vi "Build and convert part number.vi"(10 "Digit Array":T1[](array[typedef]), 11 "Unsigned Byte Array":u8[][](array[numeric])) -> (2 "Part Number Found Out":bool, 3 "Part Number Out":i32)   [LabVIEW 2023]
uses:
  Cluster Digit.ctl
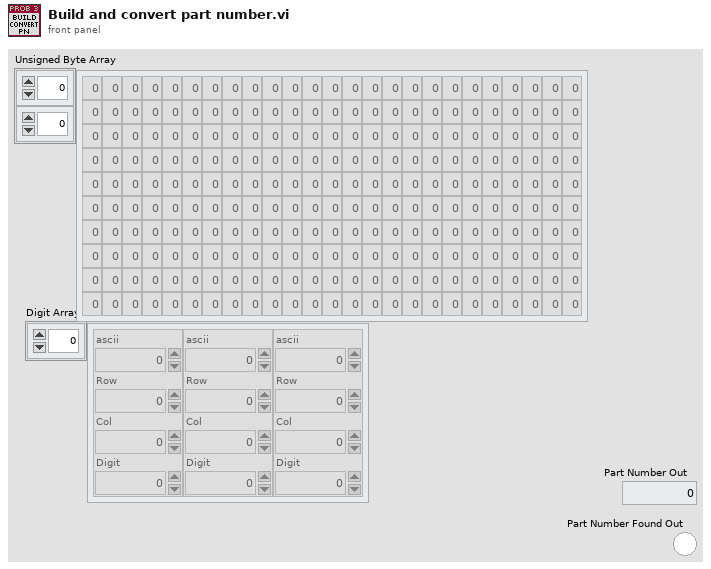
[diagram p1: front panel]
types:
  T1 = typedef "Cluster Digit.ctl" = cluster{"ascii":u8, "Row":i32, "Col":i32, "Digit":i32}
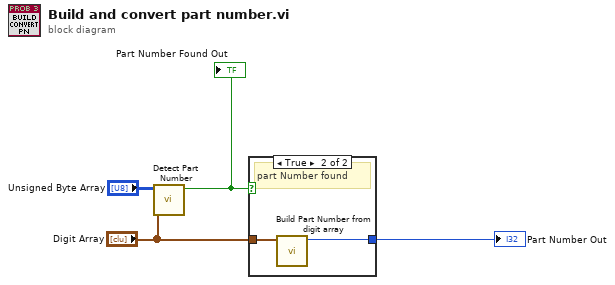
[diagram p0: block diagram]
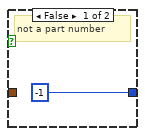
[diagram p2: hidden frame]
diagram:
  n1 = call "Detect Part Number.vi"("Digit Array"="Digit Array", "Unsigned Byte Array"="Unsigned Byte Array") -> ("Is a part Number"=w3:bool)  [unwired: 9 in]
  "Part Number Found Out" <- w3
  n2 = case shown="True" w3 {
    tunnel: [-1 ("Part Number Out") w6] -> w2
    tunnel: "Digit Array" -> [_ w7]
    frame False {
      # "not a part number"
    }
    frame True {
      # "part Number found"
      n3 = call "Build Part Number from digit array.vi"("Digit Array"=w7) -> ("Part Number Out"=w6:i32)  [unwired: 10 in]
    }
  }
  "Part Number Out" <- w2
